vi "MathCad_Wrksht_Recalc.vi"(8 "error in (no error)":errorcluster, 11 "Worksheet Reference":refnum<k7>) -> (0 "error out":errorcluster, 3 "Worksheet Reference":refnum<k7>)   [LabVIEW 2012, in "Design Server.lvlib"]
doc: "Recalculates the worksheet. Typically used after a value has been set or changed so that the worksheet can recalculate the new results\n\nInputs\nWorksheet Reference- Reference to the opened Mathcad Worksheet Class Reference outputted by the Mathcad_File_Open.vi\n\nError In -Error Cluster\n\nOutputs\nIMathcadWorksheet Reference - Reference to the opened IMathcadWorksheet Reference outputted by the Mathcad_File_Open.vi\n\nError Out- Error Cluster"
uses:
  Design Server.lvlib
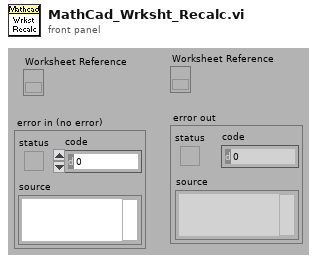
[diagram p1: front panel]
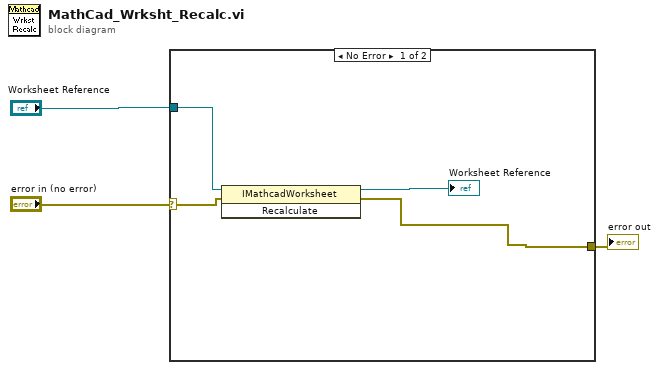
[diagram p0: block diagram]
diagram:
  n1 = case shown="No Error" "error in (no error)" {
    selector: "error in (no error)" -> [w4 w8]
    tunnel: [w6 w8] -> w3
    tunnel: "Worksheet Reference" -> [w7 _]
    frame No Error {
      n2 = invoke class="IMathcadWorksheet" method="Recalculate"(reference=w7, error in=w4) -> (reference out=→"Worksheet Reference":refnum<k7>, error out=w6:errorcluster)  [unwired: 1 in, 1 out]
    }
    frame Error {
    }
  }
  "error out" <- w3
